vi "Add Node.vi"(8 "error in (no error)":errorcluster, 10 "Node to Add":refnum<class "INode.lvclass">, 11 "dir in":refnum<class "dir.lvclass">) -> (0 "error out":errorcluster, 3 "dir out":refnum<class "dir.lvclass">)   [LabVIEW 2023, in "d7.lvlib" / "dir.lvclass"]
uses:
  dir.lvclass
  INode/INode.lvclass
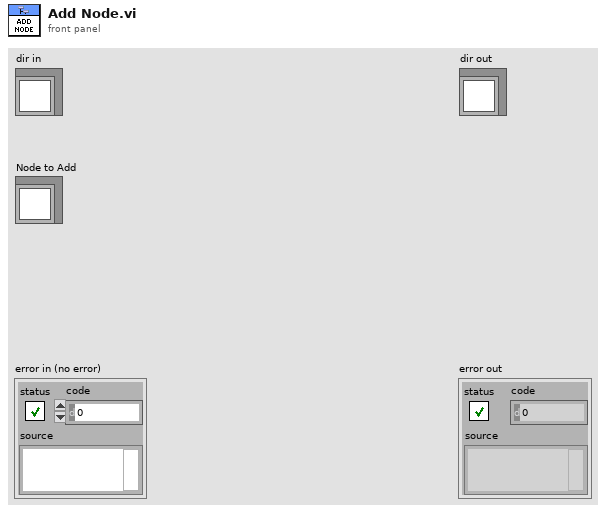
[diagram p1: front panel]
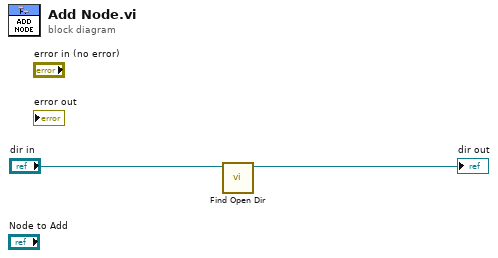
[diagram p0: block diagram]
diagram:
  n1 = call "Find Open Dir.vi"("dir in"="dir in") -> ("dir out"=→"dir out":refnum<class "dir.lvclass">)  [unwired: 8 in, 2 out]
